vi "08 - geometry rendering.vi"() -> ()   [LabVIEW 2015]
uses:
  Libraries/LibSDL2 Wrapper/Controls/Init Flags.ctl
  Libraries/LibSDL2 Wrapper/Controls/Rectangle.ctl
  Libraries/LibSDL2 Wrapper/LibSDL2.lvlib
panel:
  out "Error":string
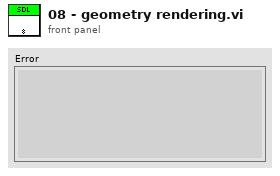
[diagram p1: front panel]
types:
  T1 = typedef "LibSDL2.lvlib/Rectangle.ctl" = cluster{"x":i32, "y":i32, "Width":i32, "Height":i32}
  T2 = typedef "LibSDL2.lvlib/Init Flags.ctl" = u32
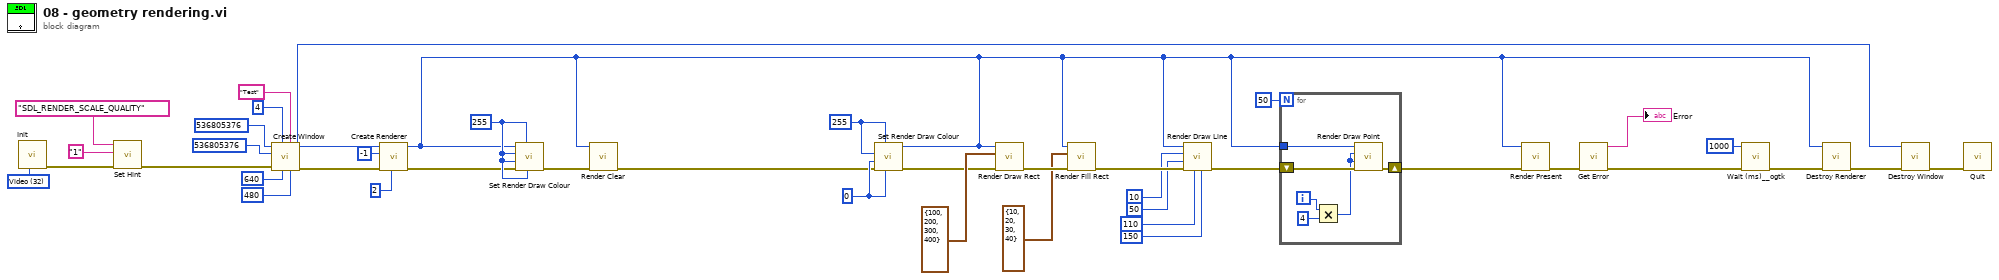
[diagram p0: block diagram]
diagram:
  w13 = u8 0 ("B")
  w15 = u8 255 ("R")
  w24 = u8 255 ("R")
  w41 = T2 32 items=["Timer"=1, "Audio"=16, "Video"=32, "Joystick"=512, "Haptic"=4096, "Game Controller"=8192, "Events"=16384, "No Parachute"=1048576, "Everything"=17244689] ("Init Flags")
  n1 = call "Init.vi"("Flags"=w41) -> ("error out"=w32:errorcluster)  [unwired: 9 in, 1 out]
  n2 = call "Set Hint.vi"("error in"=w32, "Value"="1", "Name"="SDL_RENDER_SCALE_QUALITY") -> ("error out"=w31:errorcluster)  [unwired: 7 in, 1 out]
  n3 = call "Create Window.vi"("Height"=480, "Title"="Test", "Width"=640, "Flags"=u32 4, "error in"=w31, "Position y"=u32 536805376 ("Flags"), "Position x"=u32 536805376 ("Flags")) -> ("error out"=w28:errorcluster, "Window Pointer"=w27:u32)  [unwired: 3 in]
  n4 = call "Create Renderer.vi"("Flags"=u32 2, "error in"=w28, "Index"=-1, "Window Pointer"=w27) -> ("error out"=w22:errorcluster, "Renderer Pointer"=w2:u32)  [unwired: 6 in]
  n5 = call "Set Render Draw Colour.vi"("B"=w24, "A"=w24, "error in (no error)"=w22, "G"=w24, "R"=w24, "Renderer Pointer"=w2) -> ("error out"=w18:errorcluster)  [unwired: 4 in, 1 out]
  n6 = call "Render Clear.vi"("error in"=w18, "Renderer Pointer"=w2) -> ("error out"=w12:errorcluster)  [unwired: 8 in, 1 out]
  n7 = call "Set Render Draw Colour.vi"("B"=w13, "A"=w15, "error in (no error)"=w12, "G"=w13, "R"=w15, "Renderer Pointer"=w2) -> ("error out"=w14:errorcluster)  [unwired: 4 in, 1 out]
  n8 = call "Render Draw Rect.vi"("error in"=w14, "Rectangle"=T1 {"x"=100, "y"=200, "Width"=300, "Height"=400}, "Renderer Pointer"=w2) -> ("error out"=w11:errorcluster)  [unwired: 7 in, 1 out]
  n9 = call "Render Fill Rect.vi"("error in"=w11, "Rectangle"=T1 {"x"=10, "y"=20, "Width"=30, "Height"=40}, "Renderer Pointer"=w2) -> ("error out"=w9:errorcluster)  [unwired: 7 in, 1 out]
  n10 = call "Render Draw Line.vi"("y2"=150 ("y1"), "x2"=110 ("x1"), "error in"=w9, "y1"=50, "x1"=10, "Renderer Pointer"=w2) -> ("error out"=w4:errorcluster)  [unwired: 4 in, 1 out]
  n11 = for {
    N: 50 -> [_]
    tunnel: w2 -> [w46]
    shift-right: [w45] -> w1
    shift-left: w4 -> [w47]
    i -> [w44]
    n12 = Multiply(x=w44, y=4) -> (x*y=w42:i32)
    n13 = call "Render Draw Point.vi"("error in"=w47, "y"=w42, "x"=w42, "Renderer Pointer"=w46) -> ("error out"=w45:errorcluster)  [unwired: 6 in, 1 out]
  }
  n14 = call "Render Present.vi"("error in"=w1, "Renderer Pointer"=w2) -> ("error out"=w21:errorcluster)  [unwired: 9 in]
  n15 = call "Get Error.vi"("error in"=w21) -> ("error out"=w20:errorcluster, "Error"=→"Error":string)  [unwired: 9 in]
  n16 = call <userlib>:"Wait (ms)__ogtk.vi"("error in (no error)"=w20, "milliseconds to wait"=u32 1000) -> ("error out"=w17:errorcluster)  [unwired: 8 in, 1 out]
  n17 = call "Destroy Renderer.vi"("error in"=w17, "Renderer Pointer"=w2) -> ("error out"=w23:errorcluster)  [unwired: 9 in]
  n18 = call "Destroy Window.vi"("error in"=w23, "Window Pointer"=w27) -> ("error out"=w19:errorcluster)  [unwired: 9 in]
  n19 = call "Quit.vi"("error in"=w19) -> ()  [unwired: 10 in, 1 out]
